vi "gjson_ClusterString.vi"(8 "error in":errorcluster, 10 "Cluster to Find":string, 11 "String In":string) -> (0 "error out":errorcluster, 2 "Rest":string, 3 "Cluster":string)   [LabVIEW 2015, in "Json2Labv.lvlib"]
uses:
  Json2Labv.lvlib
  <vilib>/regexp/Match Regular Expression.xnode
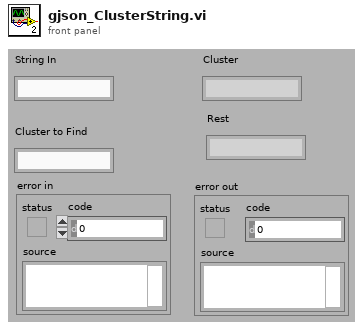
[diagram p1: front panel]
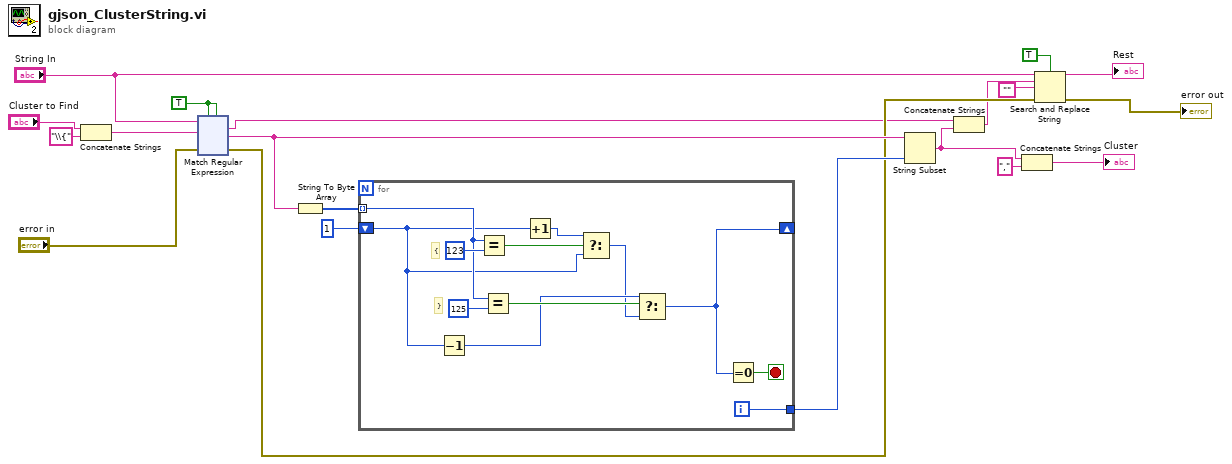
[diagram p0: block diagram]
diagram:
  w18 = TRUE ("ignore case? (F)")
  n1 = Concatenate Strings("Cluster to Find", "\\{" ("string")) -> (w15:string)
  n2 = xnode "Match Regular Expression"("input string"="String In", "regular expression"=w15, "error in"="error in", "ignore case? (F)"=w18, "multiline? (F)"=w18) -> ("whole match"=w1:string, "after match"=w11:string, "error out"=w7:errorcluster)  [unwired: 1 in, 2 out]
  n3 = String To Byte Array(string=w11) -> (unsigned byte array=w19:u8[])
  n4 = for {
    tunnel: w19 -> [w29] mode=indexing
    shift-right: [w23] -> _
    shift-left: 1 -> [w26]
    tunnel: [w21] -> w16
    i -> [w21]
    stop <- w22 stop-if-true
    # "{"
    # "}"
    n5 = Decrement(x=w26) -> (x-1=w25:i32)
    n6 = Equal?(x=w29, y=u8 123) -> (x = y?=w31:bool)
    n7 = Equal?(x=w29, y=u8 125) -> (x = y?=w27:bool)
    n8 = Increment(x=w26) -> (x+1=w30:i32)
    n9 = Select(t=w30, s=w31, f=w26) -> (s? t:f=w24:i32)
    n10 = Select(t=w25, s=w27, f=w24) -> (s? t:f=w23:i32)
    n11 = Equal To 0?(x=w23) -> (x = 0?=w22:bool)
  }
  n12 = String Subset(string=w11, length (rest)=w16) -> (substring=w3:string)  [unwired: 1 in]
  n13 = Concatenate Strings(w1, w3) -> (w2:string)
  n14 = Concatenate Strings(w3, "," ("string")) -> (→"Cluster":string)
  n15 = Search and Replace String(case sensitive?=TRUE ("replace all? (F)"), input string="String In", search string=w2, replace string="", error in=w7) -> (result string=→"Rest":string, error out=→"error out":errorcluster)  [unwired: 3 in, 2 out]
